vi "Begin.vi"() -> (0 "error out":errorcluster)   [LabVIEW 2012]
doc: "Called before other user functions, this VI is expected to open initial I/O refnums, load in file data, and do all program initialization. Notice that the <B>error out</B> terminal is simply used for data flow. Wiring it to other structures or subVIs ensures that this VI runs first."
uses:
  <vilib>/Rock Robotics/WPI/DriverStation/WPI_DriverStationRobotMode2.ctl
  <vilib>/Rock Robotics/WPI/Joystick/WPI_JoystickDeviceEnum.ctl
  <vilib>/Rock Robotics/SystemInterfaces/DIO/FPGA_DIOPWMChannel.ctl
  <vilib>/Rock Robotics/SystemInterfaces/DIO/FPGA_DIORelayChannel.ctl
  <vilib>/Rock Robotics/WPI/Relay/WPI_RelayDirection.ctl
  <vilib>/Rock Robotics/SystemInterfaces/DIO/FPGA_DIOChannel.ctl
  <vilib>/Rock Robotics/WPI/Encoder/WPI_EncoderType.ctl
  <vilib>/Rock Robotics/SystemInterfaces/AI/FPGA_AIGyroChannel.ctl
  <vilib>/Rock Robotics/WPI/Solenoid/WPI_SolenoidChannel.ctl
  <vilib>/Rock Robotics/SystemInterfaces/Typedef/FPGA_TypedefSolenoidModule.ctl
  Robot Global Data.vi
  <vilib>/Rock Robotics/WPI/RobotDrive/WPI_RobotDriveOpen4MotorWithTalon.vi
  <vilib>/Rock Robotics/WPI/Solenoid/WPI_SolenoidOpenSingle.vi
  <vilib>/Rock Robotics/WPI/Solenoid/Deprecated/WPI_SolenoidSetBool.vi
  <vilib>/Rock Robotics/WPI/Counter/WPI_CounterDigitalInputToDigitalSource.vi
  <vilib>/Rock Robotics/WPI/MotorControl/WPI_MotorControlOpen Jaguar.vi
  <vilib>/Rock Robotics/WPI/Compressor/WPI_CompressorGetSetRefNum.vi
  <vilib>/Rock Robotics/SystemInterfaces/Typedef/FPGA_TypedefDigitalModule.ctl
  <vilib>/Rock Robotics/WPI/MotorControl/WPI_MotorControlOpen Talon.vi
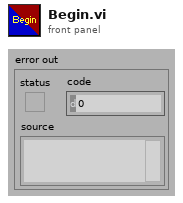
[diagram p1: front panel]
types:
  T1 = typedef "FPGA_DIOChannel.ctl" = enum8{"DIO 1", "DIO 2", "DIO 3", "DIO 4", "DIO 5", "DIO 6", "DIO 7", "DIO 8", "DIO 9", "DIO 10", "DIO 11", "DIO 12", "DIO 13", "DIO 14", "Invalid"}
  T2 = typedef "WPI_SolenoidChannel.ctl" = enum8{"Solenoid 1", "Solenoid 2", "Solenoid 3", "Solenoid 4", "Solenoid 5", "Solenoid 6", "Solenoid 7", "Solenoid 8", "Invalid"}
  T3 = typedef "FPGA_TypedefSolenoidModule.ctl" = enum16{"Solenoid Module 1", "Solenoid Module 2"}
  T4 = typedef "FPGA_AIGyroChannel.ctl" = enum8{"AI 1", "AI 2", "Invalid"}
  T5 = typedef "WPI_EncoderType.ctl" = enum16{"1x", "2x", "4x"}
  T6 = typedef "FPGA_DIORelayChannel.ctl" = enum8{"Relay 1", "Relay 2", "Relay 3", "Relay 4", "Relay 5", "Relay 6", "Relay 7", "Relay 8", "Invalid"}
  T7 = typedef "WPI_JoystickDeviceEnum.ctl" = enum16{"USB 1", "USB 2", "USB 3", "USB 4", "Kinect 1", "Kinect 2"}
  T8 = typedef "FPGA_DIOPWMChannel.ctl" = enum8{"PWM 1", "PWM 2", "PWM 3", "PWM 4", "PWM 5", "PWM 6", "PWM 7", "PWM 8", "PWM 9", "PWM 10", "Invalid"}
  T9 = typedef "WPI_RelayDirection.ctl" = enum16{"Both directions", "Forward only", "Reverse only"}
  T10 = typedef "WPI_DriverStationRobotMode2.ctl" = enum16{"Autonomous Disabled", "Autonomous Enabled", "Teleop Disabled", "Teleop Enabled", "Timeout", "Finish", "Test Disabled", "Test Enabled"}
  T11 = typedef "WPI_MotorControlDeviceRef.ctl" = cluster{"DeviceStatus":errorcluster, "Type":enum16{"PWM", "CAN"}, "PWM":cluster{"Digital Module":T12, "PWM Channel":T8, "DeadBand":T13}, "CAN":cluster{"Device Number":u8, "Control Mode":T14, "Semaphore":T15, "Max Vout":dbl}, "Invert":bool, "TransformRef":T16, "InvTransformRef":T16}
  T12 = typedef "FPGA_TypedefDigitalModule.ctl" = enum16{"Digital Module 1", "Digital Module 2"}
  T13 = typedef "WPI_PWMDeadband.ctl" = cluster{"Name":string, "maxPositivePwm":i32, "minPositivePwm":i32, "centerPwm":i32, "maxNegativePwm":i32, "minNegativePwm":i32, "angularRange":u16}
  T14 = typedef "WPI_CANJaguar_ControlMode.ctl" = enum8{"Percent VBus", "Current", "Speed", "Position", "Voltage"}
  T15 = typedef "Semaphore RefNum" = refnum<k1>
  T16 = typedef "WPI_PWMTransform_ConPane.ctl" = refnum<vi>
  T17 = typedef "WPI_DigitalInputDevRef.ctl" = cluster{"DevStatus":errorcluster, "DIO Channel":T1, "Digital Module":T12}
  T18 = typedef "WPI_ServoDeviceRef.ctl" = cluster{"DeviceStatus":errorcluster, "Digital Module":T12, "PWM Channel":T8, "DeadBand":T13}
  T19 = typedef "WPI_CompressorDevRef.ctl" = cluster{"DevStatus":errorcluster, "DigitalInputDevRef":T17, "RelayDevRef":T20}
  T20 = typedef "WPI_RelayDevRef.ctl" = cluster{"DevStatus":errorcluster, "Relay Channel":T6, "Digital Module":T12, "Relay Direction":T9}
  T21 = typedef "WPI_JoystickDevRef.ctl" = cluster{"Device":T7}
  T22 = typedef "WPI_SolenoidDevRef.ctl" = cluster{"DevStatus":errorcluster, "Solenoid Module":T3, "Forward Solenoid Channel":T2, "Reverse Solenoid Channel":T2}
  T23 = typedef "FPGA_CounterEncoderSourceConvertionLVSourceType.ctl" = cluster{"DevStatus":errorcluster, "AnalogTriggerMode?":bool, "DigitalMode":cluster{"Digital Module":T12, "DIO Channel":T24}, "AnalogTriggerMode":cluster{"AnalogTriggerIndex":T25, "OutputType":T26}}
  T24 = typedef "FPGA_DIODigitalSourceChannel.ctl" = enum8{"DIO 1", "DIO 2", "DIO 3", "DIO 4", "DIO 5", "DIO 6", "DIO 7", "DIO 8", "DIO 9", "DIO 10", "DIO 11", "DIO 12", "DIO 13", "DIO 14", "Disabled"}
  T25 = typedef "FPGA_AnalogTriggerIndex.ctl" = enum8{"Trig 0", "Trig 1", "Trig 2", "Trig 3", "Trig 4", "Trig 5", "Trig 6", "Trig 7", "Invalid"}
  T26 = typedef "FPGA_AnalogTriggerOutType.ctl" = enum16{"InWindow", "TriggerState", "Rising", "Falling"}
  T27 = typedef "WPI_GyroDevRef.ctl" = cluster{"DevStatus":errorcluster, "Analog Module":T28, "Analog Channel":T29, "Offset":dbl, "Gain (VoltsPerDegree/Second)":dbl}
  T28 = typedef "FPGA_TypedefAnalogModule.ctl" = enum16{"Analog Module 1", "Analog Module 2"}
  T29 = typedef "FPGA_AIChannel.ctl" = enum8{"AI 1", "AI 2", "AI 3", "AI 4", "AI 5", "AI 6", "AI 7", "AI 8", "Invalid"}
  T30 = typedef "WPI_RobotDriveDevRef.ctl" = cluster{"DevStatus":errorcluster, "Motors[]":T11[], "Square Inputs":bool, "Max Output":dbl, "Isochronous":bool}
  T31 = typedef "WPI_EncoderDevRef.ctl" = cluster{"DevStatus":errorcluster, "EncoderIndex":T32, "CounterIndex":T33, "DistancePerCount":dbl, "Decoding Type":T5}
  T32 = typedef "FPGA_EncoderIdx.ctl" = enum8{"Enc 0", "Enc 1", "Enc 2", "Enc 3", "Invalid"}
  T33 = typedef "FPGA_CounterCtrSystemIndex.ctl" = enum8{"Ctr 0", "Ctr 1", "Ctr 2", "Ctr 3", "Ctr 4", "Ctr 5", "Ctr 6", "Ctr 7", "Invalid"}
  T34 = cluster{"Voltage":dbl, "Target Speed":dbl, "Angle Up?":bool}
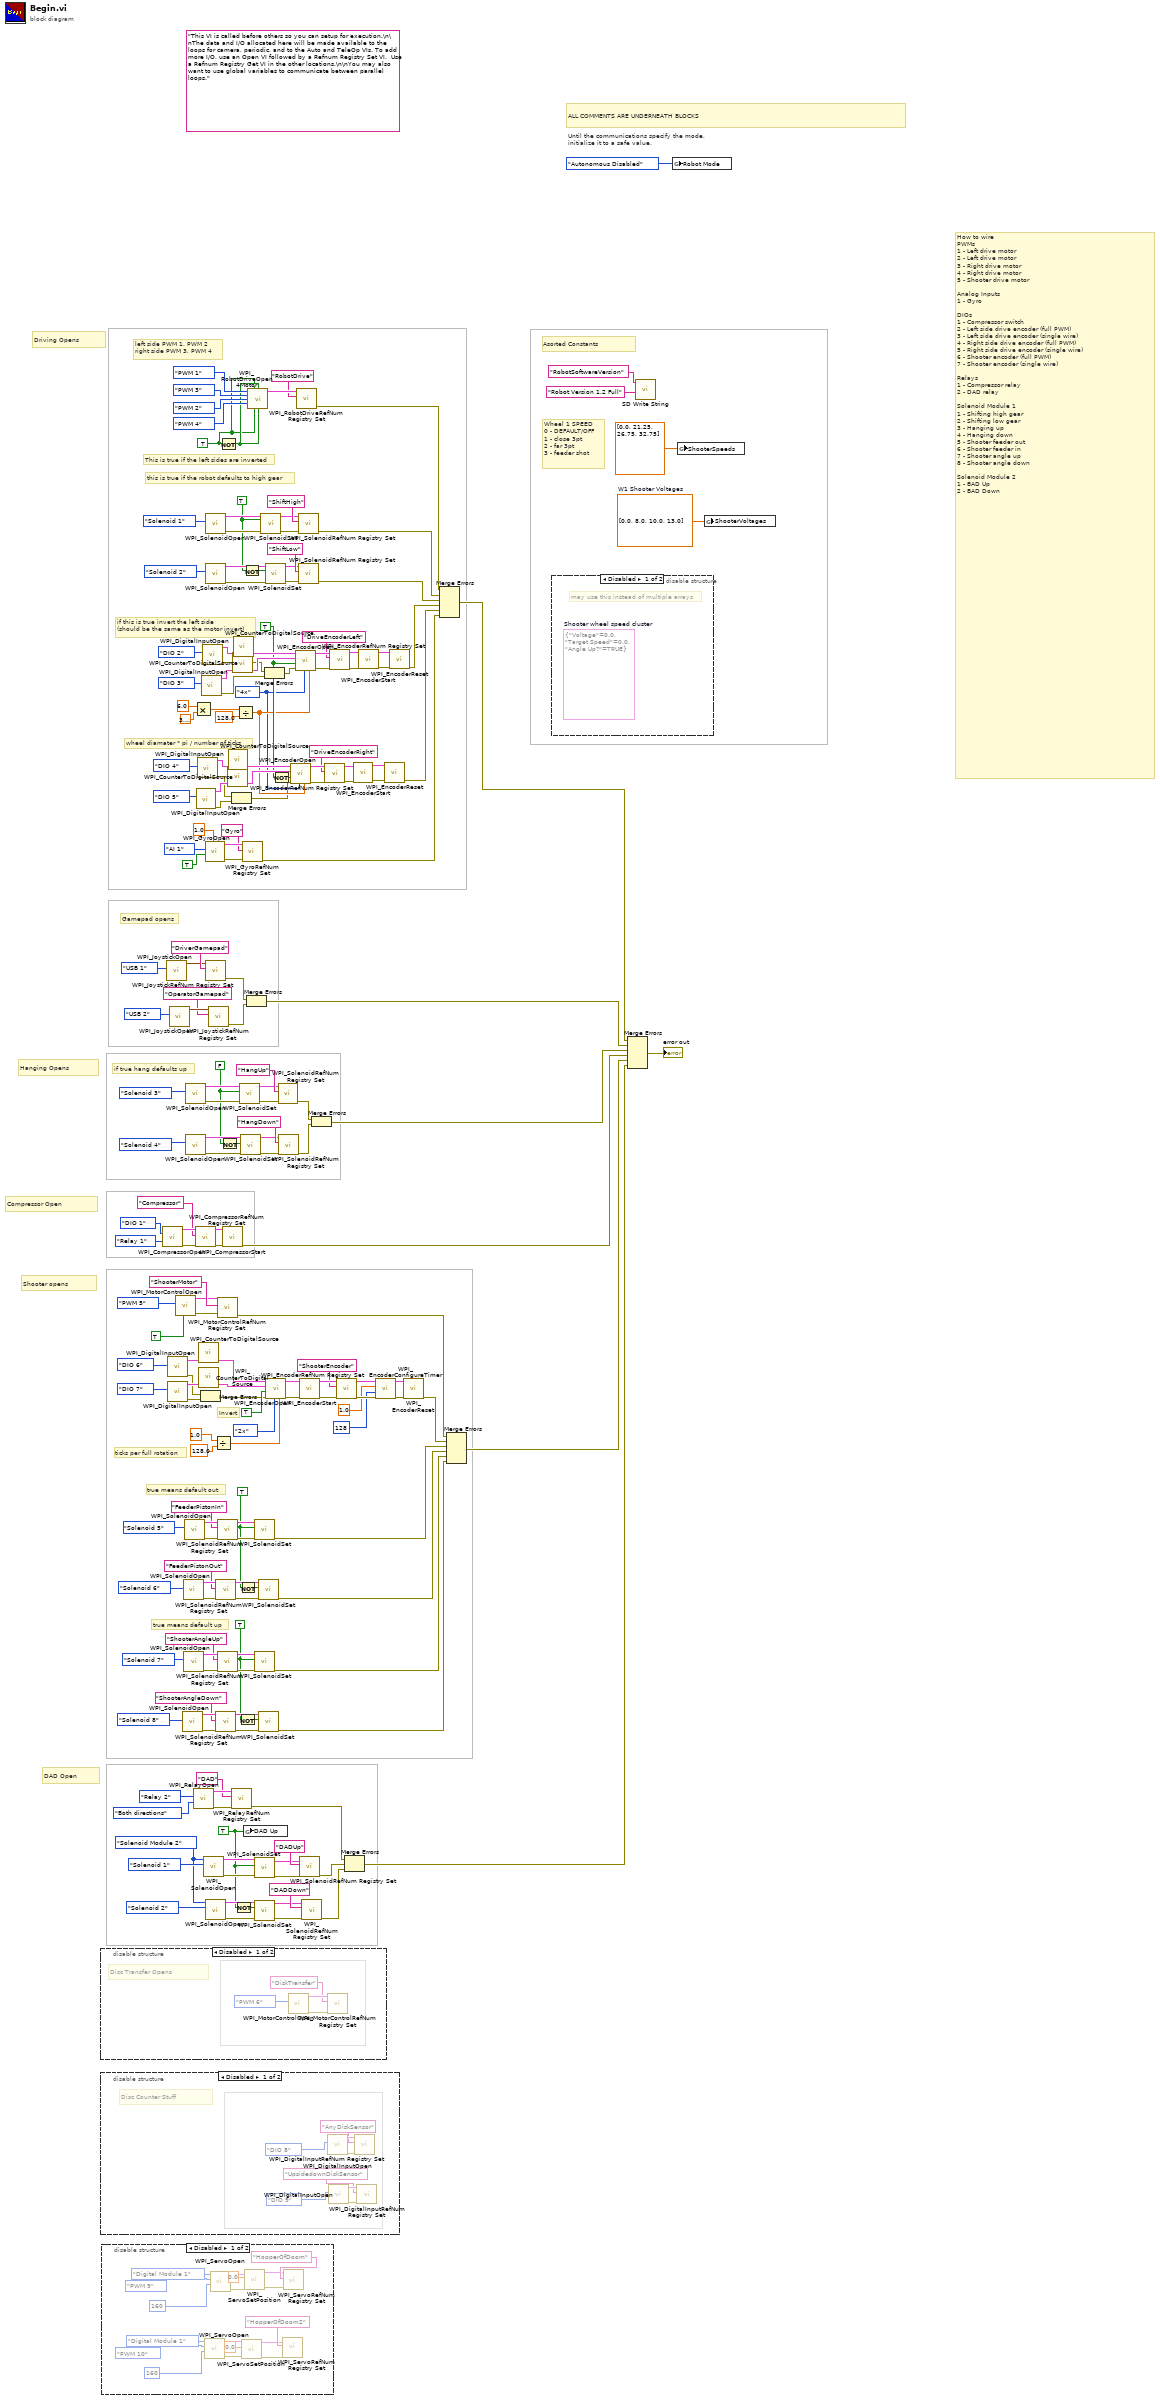
[diagram p0: block diagram]
diagram:
  w62 = TRUE
  w76 = TRUE
  w35 = TRUE
  w37 = FPGA_TypedefSolenoidModule."Solenoid Module 2" ("Solenoid Module (Module 1)")
  w38 = FALSE
  w40 = WPI_EncoderType."4x" ("Decoding Type")
  w42 = TRUE ("Invert Direction (False)")
  w144 = dbl[] [0.0, 8.0, 10.0, 13.0]  # W1 Shooter Voltages
  w60 = TRUE
  w58 = TRUE ("Rear Left Motor Inverted")
  (unwired) "This VI is called before others so you can setup for execution.\n\nThe data and I/O allocated here will be made available to the loops for camera, periodic, and to the Auto and TeleOp VIs. To add more I/O, use an Open VI followed by a Refnum Registry Set VI.  Use a Refnum Registry Get VI in the other locations.\n\nYou may also want to use global variables to communicate between parallel loops."
  # "How to wire\nPWMs\n1 - Left drive motor\n2 - Left drive motor\n3 - Right drive motor\n4 - Right drive motor\n5 - Shooter drive motor\n\nAnalog Inputs\n1 - Gyro\n\nDIOs\n1 - Compressor switch\n2 - Left side drive encoder (full PWM)\n3 - Left side drive encoder (single wire)\n4 - Right side drive encoder (full PWM)\n5 - Right side drive encoder (single wire)\n6 - Shooter encoder (full PWM)\n7 - Shooter encoder (single wire)\n\nRelays\n1 - Compressor relay\n2 - DAD relay\n\nSolenoid Module 1\n1 - Shifting high gear\n2 - Shifting low gear\n3 - Hanging up\n4 - Hanging down\n5 - Shooter feeder out\n6 - Shooter feeder in\n7 - Shooter angle up\n8 - Shooter angle down\n\nSolenoid Module 2\n1 - BAD Up\n2 - BAD Down"
  # "Asorted Constants"
  # "true means default up"
  # "true means default out"
  # "if true hang defaults up"
  # "Gamepad opens"
  # "wheel diamater * pi / number of ticks"
  # "if this is true invert the left side\n(should be the same as the motor invert)"
  # "this is true if the robot defaults to high gear"
  # "left side PWM 1, PWM 2\nright side PWM 3, PWM 4"
  # "This is true if the left sides are inverted"
  # "Compressor Open"
  # "Wheel 1 SPEED\n0 - DEFAULT/OFF\n1 - close 3pt\n2 - far 3pt\n3 - feeder shot"
  # "DAD Open"
  # "Hanging Opens"
  # "Driving Opens"
  # "Shooter opens"
  # "Invert"
  # "ticks per full rotation"
  # "ALL COMMENTS ARE UNDERNEATH BLOCKS"
  # "Until the communications specify the mode,\ninitialize it to a safe value."
  n1 = disable-structure shown="Disabled" {
    frame Disabled {
      # "Disc Transfer Opens"
      n2 = call-poly <vilib>:"WPI_MotorControlOpen.vi"("PWM Channel"=FPGA_DIOPWMChannel."PWM 6") -> ("error out"=w206:errorcluster, "MotorControlDeviceRef"=w207:T11)  [unwired: 9 in]
      n3 = call <vilib>:"WPI_MotorControlRefNum Registry Set.vi"("error in (no error)"=w206, "refnum name"="DiskTransfer", "MotorControlDevRef"=w207) -> ()  [unwired: 7 in, 2 out]
    }
    frame Enabled {
    }
  }
  n4 = disable-structure shown="Disabled" {
    frame Disabled {
      # "Disc Counter Stuff"
      n5 = call <vilib>:"WPI_DigitalInputOpen.vi"("DIO Channel"=FPGA_DIOChannel."DIO 8") -> ("error out"=w216:errorcluster, "DigitalInputDevRef"=w215:T17)  [unwired: 9 in]
      n6 = call <vilib>:"WPI_DigitalInputOpen.vi"("DIO Channel"=FPGA_DIOChannel."DIO 9") -> ("error out"=w214:errorcluster, "DigitalInputDevRef"=w213:T17)  [unwired: 9 in]
      n7 = call <vilib>:"WPI_DigitalInputRefNum Registry Set.vi"("error in (no error)"=w216, "refnum name"="AnyDiskSensor", "DigitalInputDevRef"=w215) -> ()  [unwired: 7 in, 2 out]
      n8 = call <vilib>:"WPI_DigitalInputRefNum Registry Set.vi"("error in (no error)"=w214, "refnum name"="UpsidedownDiskSensor", "DigitalInputDevRef"=w213) -> ()  [unwired: 7 in, 2 out]
    }
    frame Enabled {
    }
  }
  n9 = disable-structure shown="Disabled" {
    frame Disabled {
      n10 = call <vilib>:"WPI_ServoOpen.vi"("Angular Range"=160, "PWM Channel"=FPGA_DIOPWMChannel."PWM 10", "Digital Module (Module 1)"=FPGA_TypedefDigitalModule."Digital Module 1") -> ("error out"=w222:errorcluster, "ServoDeviceRef"=w221:T18)  [unwired: 7 in]
      n11 = call <vilib>:"WPI_ServoOpen.vi"("Angular Range"=160, "PWM Channel"=FPGA_DIOPWMChannel."PWM 9", "Digital Module (Module 1)"=FPGA_TypedefDigitalModule."Digital Module 1") -> ("error out"=w226:errorcluster, "ServoDeviceRef"=w225:T18)  [unwired: 7 in]
      n12 = call <vilib>:"WPI_ServoSetPosition.vi"("error in (no error)"=w222, "Position"=0.0, "ServoDeviceRef"=w221) -> ("error out"=w219:errorcluster, "ServoDeviceRef"=w220:T18)  [unwired: 7 in]
      n13 = call <vilib>:"WPI_ServoSetPosition.vi"("error in (no error)"=w226, "Position"=0.0, "ServoDeviceRef"=w225) -> ("error out"=w224:errorcluster, "ServoDeviceRef"=w223:T18)  [unwired: 7 in]
      n14 = call <vilib>:"WPI_ServoRefNum Registry Set.vi"("error in (no error)"=w219, "refnum name"="HopperOfDoom2", "ServoDeviceRef"=w220) -> ()  [unwired: 7 in, 2 out]
      n15 = call <vilib>:"WPI_ServoRefNum Registry Set.vi"("error in (no error)"=w224, "refnum name"="HopperOfDoom", "ServoDeviceRef"=w223) -> ()  [unwired: 7 in, 2 out]
    }
    frame Enabled {
    }
  }
  n16 = call <vilib>:"WPI_CompressorOpen.vi"("Pressure Switch DIO Channel"=FPGA_DIOChannel."DIO 1", "Relay Channel"=FPGA_DIORelayChannel."Relay 1") -> ("CompressorDevRef"=w142:T19, "error out"=w140:errorcluster)  [unwired: 12 in]
  n17 = call <vilib>:"WPI_JoystickOpen.vi"("JoystickDevice"=WPI_JoystickDeviceEnum."USB 1") -> ("JoystickDevRef"=w202:T21)  [unwired: 10 in]
  n18 = call <vilib>:"WPI_DigitalInputOpen.vi"("DIO Channel"=FPGA_DIOChannel."DIO 6") -> ("error out"=w163:errorcluster, "DigitalInputDevRef"=w177:T17)  [unwired: 9 in]
  n19 = call <vilib>:"WPI_DigitalInputOpen.vi"("DIO Channel"=FPGA_DIOChannel."DIO 7") -> ("error out"=w162:errorcluster, "DigitalInputDevRef"=w173:T17)  [unwired: 9 in]
  n20 = call <vilib>:"WPI_JoystickOpen.vi"("JoystickDevice"=WPI_JoystickDeviceEnum."USB 2") -> ("JoystickDevRef"=w146:T21)  [unwired: 10 in]
  n21 = call-poly <vilib>:"WPI_MotorControlOpen.vi"("Invert"=TRUE, "PWM Channel"=FPGA_DIOPWMChannel."PWM 5") -> ("error out"=w156:errorcluster, "MotorControlDeviceRef"=w157:T11)  [unwired: 8 in]
  n22 = call-poly <vilib>:"WPI_SolenoidOpen.vi"("Solenoid Channel"=WPI_SolenoidChannel."Solenoid 8") -> ("error out"=w72:errorcluster, "SolenoidDevRef"=w71:T22)  [unwired: 9 in]
  n23 = call-poly <vilib>:"WPI_SolenoidOpen.vi"("Solenoid Channel"=WPI_SolenoidChannel."Solenoid 6") -> ("error out"=w86:errorcluster, "SolenoidDevRef"=w85:T22)  [unwired: 9 in]
  n24 = call-poly <vilib>:"WPI_SolenoidOpen.vi"("Solenoid Channel"=WPI_SolenoidChannel."Solenoid 7") -> ("error out"=w67:errorcluster, "SolenoidDevRef"=w68:T22)  [unwired: 9 in]
  n25 = call-poly <vilib>:"WPI_SolenoidOpen.vi"("Solenoid Channel"=WPI_SolenoidChannel."Solenoid 5") -> ("error out"=w81:errorcluster, "SolenoidDevRef"=w82:T22)  [unwired: 9 in]
  n26 = call-poly <vilib>:"WPI_SolenoidOpen.vi"("Solenoid Channel"=WPI_SolenoidChannel."Solenoid 4") -> ("error out"=w108:errorcluster, "SolenoidDevRef"=w109:T22)  [unwired: 9 in]
  n27 = call-poly <vilib>:"WPI_SolenoidOpen.vi"("Solenoid Channel"=WPI_SolenoidChannel."Solenoid 3") -> ("error out"=w111:errorcluster, "SolenoidDevRef"=w110:T22)  [unwired: 9 in]
  n28 = Multiply(x=6.0, y=3.141592653589793) -> (x*y=w129:dbl)
  n29 = call <vilib>:"WPI_RelayOpen.vi"("Relay Direction"=WPI_RelayDirection."Both directions", "Relay Channel"=FPGA_DIORelayChannel."Relay 2") -> ("error out"=w180:errorcluster, "RelayDevRef"=w179:T20)  [unwired: 8 in]
  n30 = call <vilib>:"WPI_CompressorRefNum Registry Set.vi"("error in (no error)"=w140, "refnum name"="Compressor", "CompressorDevRef"=w142) -> ("error out"=w90:errorcluster, "CompressorDevRef"=w91:T19)  [unwired: 7 in]
  n31 = call <vilib>:"WPI_DigitalInputOpen.vi"("DIO Channel"=FPGA_DIOChannel."DIO 5") -> ("error out"=w28:errorcluster, "DigitalInputDevRef"=w50:T17)  [unwired: 9 in]
  n32 = call <vilib>:"WPI_DigitalInputOpen.vi"("DIO Channel"=FPGA_DIOChannel."DIO 4") -> ("error out"=w27:errorcluster, "DigitalInputDevRef"=w49:T17)  [unwired: 9 in]
  n33 = call-poly <vilib>:"WPI_CounterToDigitalSource.vi"("DigitalInputDevRef"=w177) -> ("Digital Source"=w176:T23)  [unwired: 6 in]
  n34 = call-poly <vilib>:"WPI_CounterToDigitalSource.vi"("DigitalInputDevRef"=w173) -> ("Digital Source"=w170:T23)  [unwired: 6 in]
  n35 = Merge Errors(w163, w162) -> (w164:errorcluster)
  n36 = call <vilib>:"WPI_DigitalInputOpen.vi"("DIO Channel"=FPGA_DIOChannel."DIO 3") -> ("error out"=w23:errorcluster, "DigitalInputDevRef"=w132:T17)  [unwired: 9 in]
  n37 = call <vilib>:"WPI_DigitalInputOpen.vi"("DIO Channel"=FPGA_DIOChannel."DIO 2") -> ("error out"=w24:errorcluster, "DigitalInputDevRef"=w133:T17)  [unwired: 9 in]
  n38 = call-poly <vilib>:"WPI_SolenoidOpen.vi"("Solenoid Channel"=WPI_SolenoidChannel."Solenoid 1", "Solenoid Module (Module 1)"=w37) -> ("error out"=w95:errorcluster, "SolenoidDevRef"=w99:T22)  [unwired: 8 in]
  n39 = call <vilib>:"WPI_GyroOpen.vi"("Calibration Time (s)"=1.0, "Calibrate On Open"=TRUE, "Analog Channel"=FPGA_AIGyroChannel."AI 1") -> ("error out"=w121:errorcluster, "GyroDevRef"=w120:T27)  [unwired: 6 in, 1 out]
  n40 = call-poly <vilib>:"WPI_SolenoidOpen.vi"("Solenoid Channel"=WPI_SolenoidChannel."Solenoid 1") -> ("error out"=w187:errorcluster, "SolenoidDevRef"=w190:T22)  [unwired: 9 in]
  n41 = call-poly <vilib>:"WPI_SolenoidOpen.vi"("Solenoid Channel"=WPI_SolenoidChannel."Solenoid 2") -> ("error out"=w184:errorcluster, "SolenoidDevRef"=w186:T22)  [unwired: 9 in]
  n42 = call <vilib>:"WPI_JoystickRefNum Registry Set.vi"("refnum name"="DriverGamepad", "JoystickDevRef"=w202) -> ("error out"=w20:errorcluster)  [unwired: 8 in, 1 out]
  n43 = call-poly <vilib>:"WPI_SolenoidOpen.vi"("Solenoid Channel"=WPI_SolenoidChannel."Solenoid 2", "Solenoid Module (Module 1)"=w37) -> ("error out"=w92:errorcluster, "SolenoidDevRef"=w97:T22)  [unwired: 8 in]
  n44 = call <vilib>:"WPI_JoystickRefNum Registry Set.vi"("refnum name"="OperatorGamepad", "JoystickDevRef"=w146) -> ("error out"=w19:errorcluster)  [unwired: 8 in, 1 out]
  n45 = Divide(x=1.0, y=128.0) -> (x/y=w151:dbl)
  n46 = call <vilib>:"WPI_SolenoidRefNum Registry Set.vi"("error in (no error)"=w86, "refnum name"="FeederPistonOut", "SolenoidDevRef"=w85) -> ("error out"=w88:errorcluster, "SolenoidDevRef"=w87:T22)  [unwired: 7 in]
  n47 = call <vilib>:"WPI_SolenoidRefNum Registry Set.vi"("error in (no error)"=w72, "refnum name"="ShooterAngleDown", "SolenoidDevRef"=w71) -> ("error out"=w74:errorcluster, "SolenoidDevRef"=w73:T22)  [unwired: 7 in]
  n48 = call <vilib>:"WPI_MotorControlRefNum Registry Set.vi"("error in (no error)"=w156, "refnum name"="ShooterMotor", "MotorControlDevRef"=w157) -> ("error out"=w16:errorcluster)  [unwired: 7 in, 1 out]
  n49 = call <vilib>:"WPI_SolenoidRefNum Registry Set.vi"("error in (no error)"=w81, "refnum name"="FeederPistonIn", "SolenoidDevRef"=w82) -> ("error out"=w79:errorcluster, "SolenoidDevRef"=w80:T22)  [unwired: 7 in]
  n50 = call <vilib>:"WPI_SolenoidRefNum Registry Set.vi"("error in (no error)"=w67, "refnum name"="ShooterAngleUp", "SolenoidDevRef"=w68) -> ("error out"=w65:errorcluster, "SolenoidDevRef"=w66:T22)  [unwired: 7 in]
  n51 = Not(x=w58) -> (.not. x?=w59:bool)
  n52 = Not(x=w38) -> (.not. x?=w39:bool)
  n53 = call <vilib>:"WPI_CompressorStart.vi"("error in (no error)"=w90, "CompressorDevRef"=w91) -> ("error out"=w4:errorcluster)  [unwired: 8 in, 1 out]
  n54 = call-poly <vilib>:"WPI_CounterToDigitalSource.vi"("DigitalInputDevRef"=w50) -> ("Digital Source"=w47:T23)  [unwired: 6 in]
  n55 = call-poly <vilib>:"WPI_CounterToDigitalSource.vi"("DigitalInputDevRef"=w49) -> ("Digital Source"=w45:T23)  [unwired: 6 in]
  n56 = call <vilib>:"WPI_RelayRefNum Registry Set.vi"("error in (no error)"=w180, "refnum name"="DAD", "RelayDevRef"=w179) -> ("error out"=w10:errorcluster)  [unwired: 7 in, 1 out]
  n57 = Merge Errors(w27, w28) -> (w26:errorcluster)
  n58 = call-poly <vilib>:"WPI_CounterToDigitalSource.vi"("DigitalInputDevRef"=w132) -> ("Digital Source"=w135:T23)  [unwired: 6 in]
  n59 = call-poly <vilib>:"WPI_CounterToDigitalSource.vi"("DigitalInputDevRef"=w133) -> ("Digital Source"=w137:T23)  [unwired: 6 in]
  n60 = Not(x=w35) -> (.not. x?=w36:bool)
  n61 = Divide(x=w129, y=128.0 ("x")) -> (x/y=w41:dbl)
  n62 = Not(x=w62) -> (.not. x?=w75:bool)
  n63 = Not(x=w76) -> (.not. x?=w89:bool)
  n64 = call-poly <vilib>:"WPI_SolenoidSet.vi"("error in (no error)"=w111, "Value"=w38, "SolenoidDevRef"=w110) -> ("error out"=w104:errorcluster, "SolenoidDevRef"=w107:T22)  [unwired: 7 in]
  n65 = call-poly <vilib>:"WPI_SolenoidSet.vi"("error in (no error)"=w108, "Value"=w39, "SolenoidDevRef"=w109) -> ("error out"=w105:errorcluster, "SolenoidDevRef"=w106:T22)  [unwired: 7 in]
  n66 = Not(x=w60) -> (.not. x?=w61:bool)
  n67 = call <vilib>:"WPI_GyroRefNum Registry Set.vi"("error in (no error)"=w121, "refnum name"="Gyro", "GyroDevRef"=w120) -> ("error out"=w21:errorcluster)  [unwired: 7 in, 1 out]
  n68 = global write "Robot Global Data.vi" "DAD Up"(w35) -> ()
  n69 = Merge Errors(w20, w19) -> (w6:errorcluster)
  n70 = call-poly <vilib>:"WPI_RobotDriveOpen4Motor.vi"("Rear Left Motor"=FPGA_DIOPWMChannel."PWM 1", "Rear Left Motor Inverted"=w58, "Rear Right Motor Inverted"=w59, "Rear Right Motor"=FPGA_DIOPWMChannel."PWM 3", "Front Left Motor"=FPGA_DIOPWMChannel."PWM 2", "Front Right Motor"=FPGA_DIOPWMChannel."PWM 4" ("Front Left Motor"), "Front Left Motor Inverted"=w58, "Front Right Motor Inverted"=w59) -> ("RobotDriveDevRef"=w196:T30)  [unwired: 6 in, 1 out]
  n71 = call-poly <vilib>:"WPI_SolenoidSet.vi"("error in (no error)"=w65, "Value"=w62, "SolenoidDevRef"=w66) -> ("error out"=w12:errorcluster)  [unwired: 7 in, 1 out]
  n72 = call-poly <vilib>:"WPI_SolenoidSet.vi"("error in (no error)"=w95, "Value"=w35, "SolenoidDevRef"=w99) -> ("error out"=w94:errorcluster, "SolenoidDevRef"=w98:T22)  [unwired: 7 in]
  n73 = call-poly <vilib>:"WPI_SolenoidSet.vi"("error in (no error)"=w92, "Value"=w36, "SolenoidDevRef"=w97) -> ("error out"=w93:errorcluster, "SolenoidDevRef"=w96:T22)  [unwired: 7 in]
  n74 = call-poly <vilib>:"WPI_SolenoidSet.vi"("error in (no error)"=w79, "Value"=w76, "SolenoidDevRef"=w80) -> ("error out"=w14:errorcluster)  [unwired: 7 in, 1 out]
  n75 = call-poly <vilib>:"WPI_SolenoidSet.vi"("error in (no error)"=w74, "Value"=w75, "SolenoidDevRef"=w73) -> ("error out"=w11:errorcluster)  [unwired: 7 in, 1 out]
  n76 = call-poly <vilib>:"WPI_SolenoidSet.vi"("error in (no error)"=w88, "Value"=w89, "SolenoidDevRef"=w87) -> ("error out"=w13:errorcluster)  [unwired: 7 in, 1 out]
  n77 = call-poly <vilib>:"WPI_SolenoidSet.vi"("error in (no error)"=w187, "Value"=w60, "SolenoidDevRef"=w190) -> ("error out"=w188:errorcluster, "SolenoidDevRef"=w189:T22)  [unwired: 7 in]
  n78 = Merge Errors(w24, w23) -> (w25:errorcluster)
  n79 = call-poly <vilib>:"WPI_SolenoidSet.vi"("error in (no error)"=w184, "Value"=w61, "SolenoidDevRef"=w186) -> ("error out"=w183:errorcluster, "SolenoidDevRef"=w185:T22)  [unwired: 7 in]
  n80 = call <vilib>:"WPI_EncoderOpen.vi"("DistancePerCount"=w151, "Decoding Type"=WPI_EncoderType."2x", "error in (no error)"=w164, "Invert Direction (False)"=TRUE, "BSource"=w170, "ASource"=w176) -> ("error out"=w165:errorcluster, "EncoderDevRef"=w166:T31)  [unwired: 4 in]
  n81 = Not(x=w42) -> (.not. x?=w43:bool)
  n82 = call <vilib>:"WPI_SolenoidRefNum Registry Set.vi"("error in (no error)"=w104, "refnum name"="HangUp", "SolenoidDevRef"=w107) -> ("error out"=w18:errorcluster)  [unwired: 7 in, 1 out]
  n83 = call <vilib>:"WPI_SolenoidRefNum Registry Set.vi"("error in (no error)"=w105, "refnum name"="HangDown", "SolenoidDevRef"=w106) -> ("error out"=w17:errorcluster)  [unwired: 7 in, 1 out]
  n84 = call <vilib>:"WPI_EncoderOpen.vi"("DistancePerCount"=w41, "Decoding Type"=w40, "error in (no error)"=w26, "Invert Direction (False)"=w43, "BSource"=w47, "ASource"=w45) -> ("error out"=w51:errorcluster, "EncoderDevRef"=w52:T31)  [unwired: 4 in]
  n85 = call <vilib>:"WPI_EncoderOpen.vi"("DistancePerCount"=w41, "Decoding Type"=w40, "error in (no error)"=w25, "Invert Direction (False)"=w42, "BSource"=w135, "ASource"=w137) -> ("error out"=w128:errorcluster, "EncoderDevRef"=w127:T31)  [unwired: 4 in]
  n86 = call <vilib>:"WPI_RobotDriveRefNum Registry Set.vi"("refnum name"="RobotDrive", "RobotDriveDevRef"=w196) -> ("error out"=w32:errorcluster)  [unwired: 8 in, 1 out]
  n87 = call <vilib>:"WPI_SolenoidRefNum Registry Set.vi"("error in (no error)"=w188, "refnum name"="ShiftHigh", "SolenoidDevRef"=w189) -> ("error out"=w31:errorcluster)  [unwired: 7 in, 1 out]
  n88 = call <vilib>:"WPI_SolenoidRefNum Registry Set.vi"("error in (no error)"=w183, "refnum name"="ShiftLow", "SolenoidDevRef"=w185) -> ("error out"=w30:errorcluster)  [unwired: 7 in, 1 out]
  n89 = call <vilib>:"WPI_EncoderStart.vi"("error in (no error)"=w165, "EncoderDevRef"=w166) -> ("error out"=w161:errorcluster, "EncoderDevRef"=w167:T31)  [unwired: 8 in]
  n90 = call <vilib>:"WPI_SolenoidRefNum Registry Set.vi"("error in (no error)"=w94, "refnum name"="DADUp", "SolenoidDevRef"=w98) -> ("error out"=w9:errorcluster)  [unwired: 7 in, 1 out]
  n91 = call <vilib>:"WPI_SolenoidRefNum Registry Set.vi"("error in (no error)"=w93, "refnum name"="DADDown", "SolenoidDevRef"=w96) -> ("error out"=w8:errorcluster)  [unwired: 7 in, 1 out]
  n92 = Merge Errors(w18, w17) -> (w5:errorcluster)
  n93 = call <vilib>:"WPI_EncoderRefNum Registry Set.vi"("error in (no error)"=w51, "refnum name"="DriveEncoderRight", "EncoderDevRef"=w52) -> ("error out"=w53:errorcluster, "EncoderDevRef"=w54:T31)  [unwired: 7 in]
  n94 = call <vilib>:"WPI_EncoderRefNum Registry Set.vi"("error in (no error)"=w128, "refnum name"="DriveEncoderLeft", "EncoderDevRef"=w127) -> ("error out"=w126:errorcluster, "EncoderDevRef"=w125:T31)  [unwired: 7 in]
  n95 = call <vilib>:"WPI_EncoderRefNum Registry Set.vi"("error in (no error)"=w161, "refnum name"="ShooterEncoder", "EncoderDevRef"=w167) -> ("error out"=w152:errorcluster, "EncoderDevRef"=w153:T31)  [unwired: 7 in]
  n96 = Merge Errors(w10, w9, w8) -> (w2:errorcluster)
  n97 = call <vilib>:"WPI_EncoderStart.vi"("error in (no error)"=w53, "EncoderDevRef"=w54) -> ("error out"=w55:errorcluster, "EncoderDevRef"=w56:T31)  [unwired: 8 in]
  n98 = call <vilib>:"WPI_EncoderStart.vi"("error in (no error)"=w126, "EncoderDevRef"=w125) -> ("error out"=w124:errorcluster, "EncoderDevRef"=w123:T31)  [unwired: 8 in]
  n99 = call <vilib>:"WPI_EncoderConfigureTimer.vi"("error in (no error)"=w152, "Number Samples to Average"=u8 128, "Minimum Rate"=1.0, "EncoderDevRef"=w153) -> ("error out"=w155:errorcluster, "EncoderDevRef"=w154:T31)  [unwired: 6 in]
  n100 = call <vilib>:"WPI_EncoderReset.vi"("error in (no error)"=w55, "EncoderDevRef"=w56) -> ("error out"=w22:errorcluster)  [unwired: 8 in, 1 out]
  n101 = call <vilib>:"WPI_EncoderReset.vi"("error in (no error)"=w124, "EncoderDevRef"=w123) -> ("error out"=w29:errorcluster)  [unwired: 8 in, 1 out]
  n102 = call <vilib>:"WPI_EncoderReset.vi"("error in (no error)"=w155, "EncoderDevRef"=w154) -> ("error out"=w15:errorcluster)  [unwired: 8 in, 1 out]
  n103 = Merge Errors(w32, w31, w30, w29, w22, w21) -> (w7:errorcluster)
  n104 = Merge Errors(w16, w15, w14, w13, w12, w11) -> (w3:errorcluster)
  n105 = disable-structure shown="Disabled" {
    frame Disabled {
      (unwired) T34 {"Voltage"=0.0, "Target Speed"=0.0, "Angle Up?"=TRUE}  # Shooter wheel speed cluster
      # "may use this instead of multiple arrays"
    }
    frame Enabled {
    }
  }
  n106 = Merge Errors(w7, w6, w5, w4, w3, w2) -> (→"error out":errorcluster)
  n107 = call <vilib>:"SD Write String.vi"("String"="Robot Version 1.2 Full", "Name"="RobotSoftwareVersion") -> ()  [unwired: 8 in, 2 out]
  n108 = global write "Robot Global Data.vi" "Robot Mode"(WPI_DriverStationRobotMode2."Autonomous Disabled" ("Robot Mode")) -> ()
  n109 = global write "Robot Global Data.vi" "ShooterSpeeds"(dbl[] [0.0, 21.25, 26.75, 32.75]) -> ()
  n110 = global write "Robot Global Data.vi" "ShooterVoltages"(w144) -> ()
